vi "CMN_CombineErrors.vi"(8 "Errors":errorcluster[](array[cluster])) -> (0 "error out":errorcluster)   [LabVIEW 2016]
panel:
  in  "no error":errorcluster
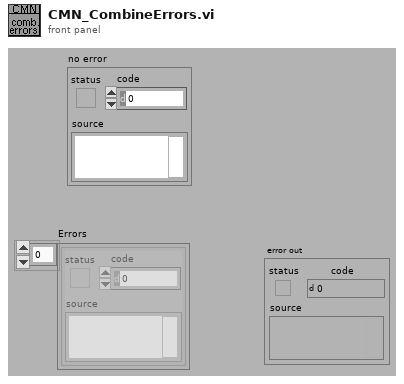
[diagram p1: front panel]
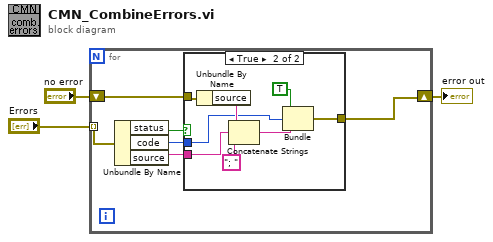
[diagram p0: block diagram]
diagram:
  n1 = for {
    tunnel: "Errors" -> [w9] mode=indexing
    shift-right: [w4] -> w1
    shift-left: "no error" -> [w7]
    n2 = Unbundle By Name(w9) -> ("status"=w8:bool, "code"=w5:i32, "source"=w6:string)
    n3 = case shown="True" w8 {
      tunnel: w7 -> [w10 w14]
      tunnel: w6 -> [_ w18]
      tunnel: w5 -> [_ w11]
      tunnel: [w10 w15] -> w4
      frame False {
      }
      frame True {
        n4 = Unbundle By Name(w14) -> ("source"=w13:string)
        n5 = Concatenate Strings(w13, w18, "; ") -> (w16:string)
        n6 = Bundle(TRUE, "code"=w11, w16) -> (w15:cluster{bool, "code":i32, string})  [unwired: 1 out]
      }
    }
  }
  "error out" <- w1
